vi "read raw commands.vi"(8 "error in":errorcluster, 11 "profibus reference":T1) -> (0 "error out":errorcluster, 2 "Data":u32[](array[numeric]), 3 "profibus reference out":T1)   [LabVIEW 2013, in "dynamic profibus.lvlib"]
uses:
  dynamic profibus.lvlib
  fpga reference.ctl
  <vilib>/rvi/interface/common/niFpgaWaitOnOcc.vi
  <vilib>/Utility/error.llb/Error Cluster From Error Code.vi
  <vilib>/rvi/errors/niLvFpgaAdjustHostInterfaceError.vi
  <vilib>/rvi/interface/nirviMethod/nirviMethod.xnode
  <vilib>/FPGAPlugInAG/Dynamic/niLvFpga_ReadFifo_Dynamic.vi
  <vilib>/rvi/errors/niLvFpgaMergeErrorWithErrorCode.vi
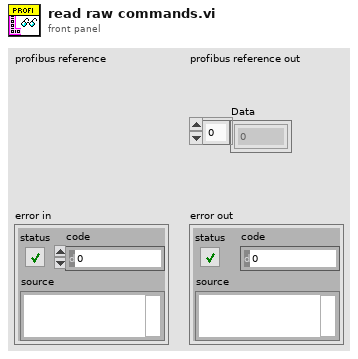
[diagram p1: front panel]
types:
  T1 = typedef "dynamic profibus.lvlib/fpga reference.ctl" = refnum<k20>
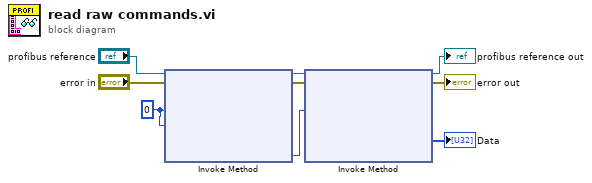
[diagram p0: block diagram]
diagram:
  w1 = u32 0 ("Number of Elements")
  n1 = xnode "Invoke Method"("FPGA VI Reference In"="profibus reference", "error in"="error in", "Number of Elements"=w1, "Timeout (ms)"=w1) -> ("FPGA VI Reference Out"=w3:T1, "error out"=w4:errorcluster, "Elements Remaining"=w2:u32)  [unwired: 1 out]
  n2 = xnode "Invoke Method"("FPGA VI Reference In"=w3, "error in"=w4, "Number of Elements"=w2) -> ("FPGA VI Reference Out"=→"profibus reference out":T1, "error out"=→"error out":errorcluster, "Data"=→"Data":u32[])  [unwired: 1 in, 1 out]
